vi "IIR_block_fast18_reg_rnd.vi"(0 "IQ_Data_In":T1, 1 "enable":bool, 7 "Decimation Factor (-1)":fxp<+,4,4> format="%#_3g", 9 "Valid In":bool, 12 "IIR 2 coeffs":T2={"b0"=0.015777587890625, "b1"=-0.030517578125, "-a1"=1.9578399658203125, "-a2"=-0.9589080810546875}) -> (4 "IQ_Data_Out":T1, 10 "output valid":bool)   [LabVIEW 2018]
uses:
  Controls/IIR_Coeffs.ctl
  <instrlib>/_niInstr/DSP/v1/Shared/Public/IQ Data.ctl
  <instrlib>/_niInstr/DSP/v1/Shared/niInstr DSP v1 Shared.lvlib
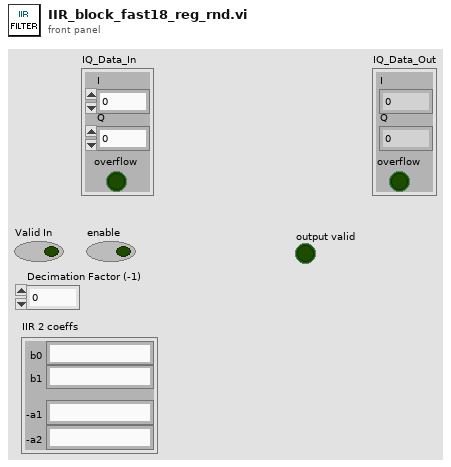
[diagram p1: front panel]
types:
  T1 = typedef "niInstr DSP v1 Shared.lvlib/IQ Data.ctl" = cluster{"I":fxp<+/-,18,1>, "Q":fxp<+/-,18,1>, "overflow":bool}
  T2 = typedef "IIR_Coeffs.ctl" = cluster{"b0":fxp<+/-,18,2>, "b1":fxp<+/-,18,2>, "-a1":fxp<+/-,18,2>, "-a2":fxp<+/-,18,2>}
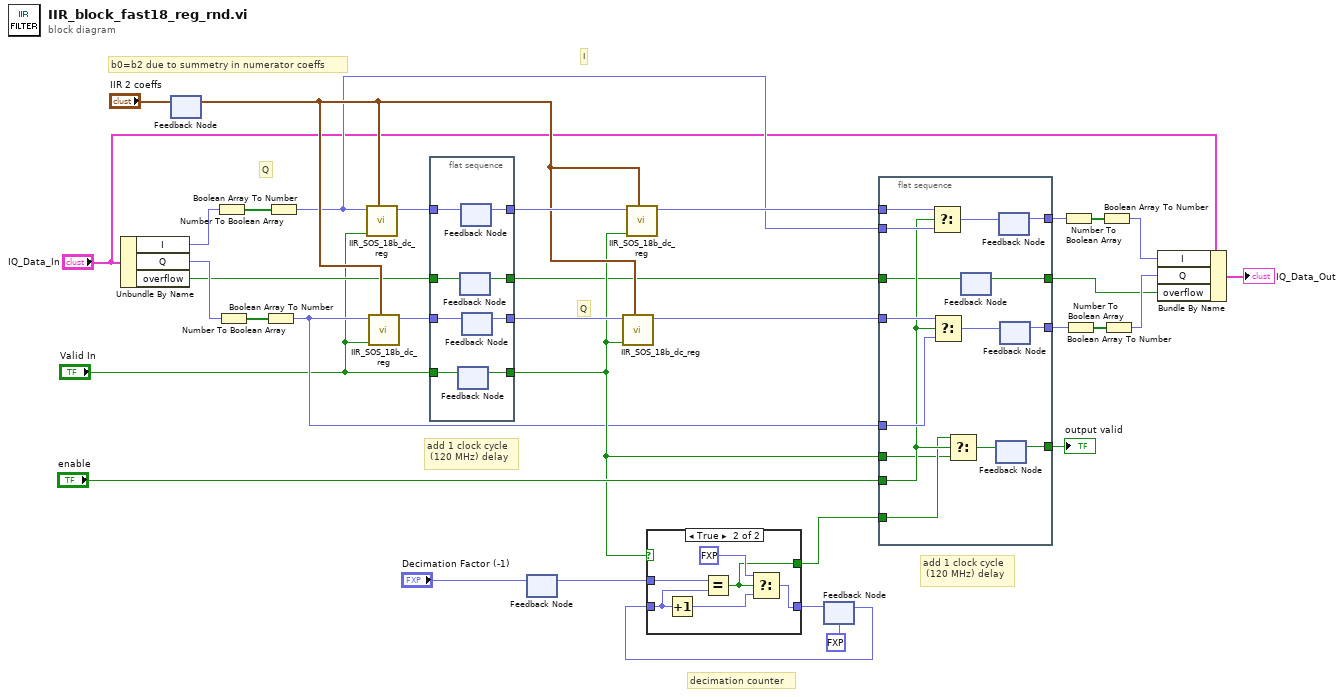
[diagram p0: block diagram]
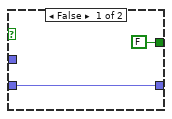
[diagram p2: hidden frame]
diagram:
  # "decimation counter"
  # "add 1 clock cycle\n (120 MHz) delay"
  # "Q"
  # "I"
  # "add 1 clock cycle\n (120 MHz) delay"
  # "Q"
  # "b0=b2 due to summetry in numerator coeffs"
  n1 = Unbundle By Name("IQ_Data_In") -> ("I"=w17:fxp<+/-,18,1>, "Q"=w14:fxp<+/-,18,1>, "overflow"=w12:bool)
  n2 = feedback #1() -> (w21:T2)  [unwired: 1 out]
  n3 = feedback-in #1("IIR 2 coeffs") -> ()
  n4 = Number To Boolean Array(number=w17) -> (Boolean array=w16:bool[])
  n5 = Number To Boolean Array(number=w14) -> (Boolean array=w13:bool[])
  n6 = Boolean Array To Number(Boolean array=w13) -> (number=w15:fxp<+/-,18,16>)
  n7 = Boolean Array To Number(Boolean array=w16) -> (number=w18:fxp<+/-,18,16>)
  n8 = call "IIR_SOS_18b_dc_reg.vi"("Coeffs SOS"=w21, "enable"="Valid In", "In SOS"=w18) -> ("out SOS"=w24:fxp<+/-,18,16>)  [unwired: 8 in]
  n9 = call "IIR_SOS_18b_dc_reg.vi"("Coeffs SOS"=w21, "enable"="Valid In", "In SOS"=w15) -> ("out SOS"=w27:fxp<+/-,18,16>)  [unwired: 8 in]
  n10 = flat-sequence {
    tunnel: w24 -> [w43]
    tunnel: [w42] -> w23
    tunnel: [w41] -> w26
    tunnel: "Valid In" -> [w40]
    tunnel: [w39] -> w19
    tunnel: w27 -> [w38]
    tunnel: w12 -> [w37]
    tunnel: [w36] -> w11
    frame #0 {
      n11 = feedback #2() -> (w39:bool)  [unwired: 1 out]
      n12 = feedback-in #2(w40) -> ()
      n13 = feedback #3() -> (w36:bool)  [unwired: 1 out]
      n14 = feedback-in #3(w37) -> ()
      n15 = feedback #4() -> (w42:fxp<+/-,18,16>)  [unwired: 1 out]
      n16 = feedback-in #4(w43) -> ()
      n17 = feedback #5() -> (w41:fxp<+/-,18,16>)  [unwired: 1 out]
      n18 = feedback-in #5(w38) -> ()
    }
  }
  n19 = feedback #6() -> (w29:fxp<+,4,4>)  [unwired: 1 in]
  n20 = feedback-in #6("Decimation Factor (-1)") -> ()
  n21 = call "IIR_SOS_18b_dc_reg.vi"("Coeffs SOS"=w21, "enable"=w19, "In SOS"=w26) -> ("out SOS"=w25:fxp<+/-,18,16>)  [unwired: 8 in]
  n22 = call "IIR_SOS_18b_dc_reg.vi"("Coeffs SOS"=w21, "enable"=w19, "In SOS"=w23) -> ("out SOS"=w22:fxp<+/-,18,16>)  [unwired: 8 in]
  n23 = feedback #7(fxp<+,4,4> 0.0 ("Mux Sel")) -> (w31:fxp<+,4,4>)
  n24 = case shown="True" w19 {
    tunnel: w31 -> [w45 w47]
    tunnel: [w45 w49] -> w32
    tunnel: [FALSE w48] -> w20
    tunnel: w29 -> [_ w46]
    frame False {
    }
    frame True {
      n25 = Increment(x=w47) -> (x+1=w50:fxp<+,4,4>)
      n26 = Equal?(x=w46, y=w47) -> (x = y?=w48:bool)
      n27 = Select(t=fxp<+,4,4> 0.0 ("Mux Sel"), s=w48, f=w50) -> (s? t:f=w49:fxp<+,4,4>)
    }
  }
  n28 = feedback-in #7(w32) -> ()
  n29 = flat-sequence {
    tunnel: w22 -> [w62]
    tunnel: [w66] -> w5
    tunnel: w25 -> [w59]
    tunnel: [w65] -> w10
    tunnel: [w64] -> w35
    tunnel: w19 -> [w55]
    tunnel: w18 -> [w63]
    tunnel: "enable" -> [w57]
    tunnel: w15 -> [w60]
    tunnel: w20 -> [w56]
    tunnel: w11 -> [w53]
    tunnel: [w52] -> w3
    frame #0 {
      n30 = Select(t=w62, s=w57, f=w63) -> (s? t:f=w61:fxp<+/-,18,16>)
      n31 = Select(t=w59, s=w57, f=w60) -> (s? t:f=w58:fxp<+/-,18,16>)
      n32 = Select(t=w56, s=w57, f=w55) -> (s? t:f=w54:bool)
      n33 = feedback #8() -> (w52:bool)  [unwired: 1 out]
      n34 = feedback-in #8(w53) -> ()
      n35 = feedback #9() -> (w64:bool)  [unwired: 1 out]
      n36 = feedback-in #9(w54) -> ()
      n37 = feedback #10() -> (w66:fxp<+/-,18,16>)  [unwired: 1 out]
      n38 = feedback-in #10(w61) -> ()
      n39 = feedback #11() -> (w65:fxp<+/-,18,16>)  [unwired: 1 out]
      n40 = feedback-in #11(w58) -> ()
    }
  }
  n41 = Number To Boolean Array(number=w5) -> (Boolean array=w6:bool[])
  n42 = Number To Boolean Array(number=w10) -> (Boolean array=w8:bool[])
  n43 = Boolean Array To Number(Boolean array=w6) -> (number=w4:fxp<+/-,18,1>)
  n44 = Boolean Array To Number(Boolean array=w8) -> (number=w7:fxp<+/-,18,1>)
  n45 = Bundle By Name(cluster="IQ_Data_In", "I"=w4, "Q"=w7, "overflow"=w3) -> (→"IQ_Data_Out":T1)
  "output valid" <- w35
